vi "change samples for test.vi"(10 "channels in":T1) -> (2 "output cluster":T1)   [LabVIEW 2020]
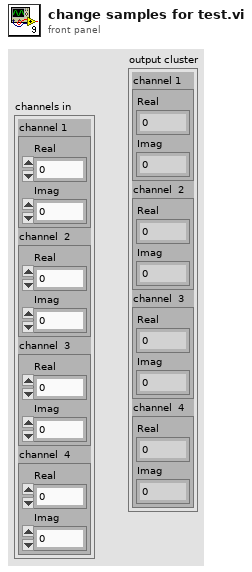
[diagram p1: front panel]
types:
  T1 = cluster{"channel 1 ":cluster{"Real":fxp<+/-,16,3>, "Imag":fxp<+/-,16,3>}, "channel  2":cluster{"Real":fxp<+/-,16,3>, "Imag":fxp<+/-,16,3>}, "channel  3":cluster{"Real":fxp<+/-,16,3>, "Imag":fxp<+/-,16,3>}, "channel  4":cluster{"Real":fxp<+/-,16,3>, "Imag":fxp<+/-,16,3>}}
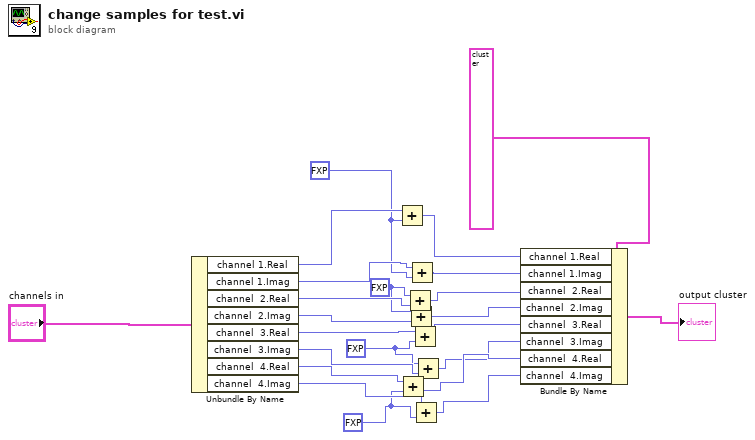
[diagram p0: block diagram]
diagram:
  w2 = fxp<+/-,25,4> 2.0 ("x")
  w14 = fxp<+/-,25,4> 1.0 ("x")
  w7 = fxp<+/-,25,4> 3.0 ("y")
  w18 = fxp<+/-,25,4> 0.0 ("y")
  n1 = Unbundle By Name("channels in") -> ("channel 1.Real"=w23:fxp<+/-,16,3>, "channel 1.Imag"=w19:fxp<+/-,16,3>, "channel  2.Real"=w16:fxp<+/-,16,3>, "channel  2.Imag"=w13:fxp<+/-,16,3>, "channel  3.Real"=w3:fxp<+/-,16,3>, "channel  3.Imag"=w6:fxp<+/-,16,3>, "channel  4.Real"=w8:fxp<+/-,16,3>, "channel  4.Imag"=w11:fxp<+/-,16,3>)
  n2 = Add(x=w23, y=w18) -> (x+y=w22:fxp<+/-,16,3>)
  n3 = Add(x=w8, y=w7) -> (x+y=w9:fxp<+/-,16,3>)
  n4 = Add(x=w14, y=w16) -> (x+y=w15:fxp<+/-,16,3>)
  n5 = Add(x=w14, y=w13) -> (x+y=w12:fxp<+/-,16,3>)
  n6 = Add(x=w19, y=w18) -> (x+y=w17:fxp<+/-,16,3>)
  n7 = Add(x=w3, y=w2) -> (x+y=w4:fxp<+/-,16,3>)
  n8 = Add(x=w11, y=w7) -> (x+y=w10:fxp<+/-,16,3>)
  n9 = Add(x=w2, y=w6) -> (x+y=w5:fxp<+/-,16,3>)
  n10 = Bundle By Name(cluster=T1 {"channel 1 "={"Real"=0.0, "Imag"=0.0}, "channel  2"={"Real"=0.0, "Imag"=0.0}, "channel  3"={"Real"=0.0, "Imag"=0.0}, "channel  4"={"Real"=0.0, "Imag"=0.0}} ("channels in"), "channel 1.Real"=w22, "channel 1.Imag"=w17, "channel  2.Real"=w15, "channel  2.Imag"=w12, "channel  3.Real"=w4, "channel  3.Imag"=w5, "channel  4.Real"=w9, "channel  4.Imag"=w10) -> (→"output cluster":T1)
